vi "example.vi"() -> ()   [LabVIEW 2016]
panel:
  in  "Stream Write":i32
  out "Stream Writer Loop readback":i32
  out "Stream Reader":i32
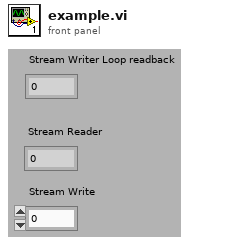
[diagram p1: front panel]
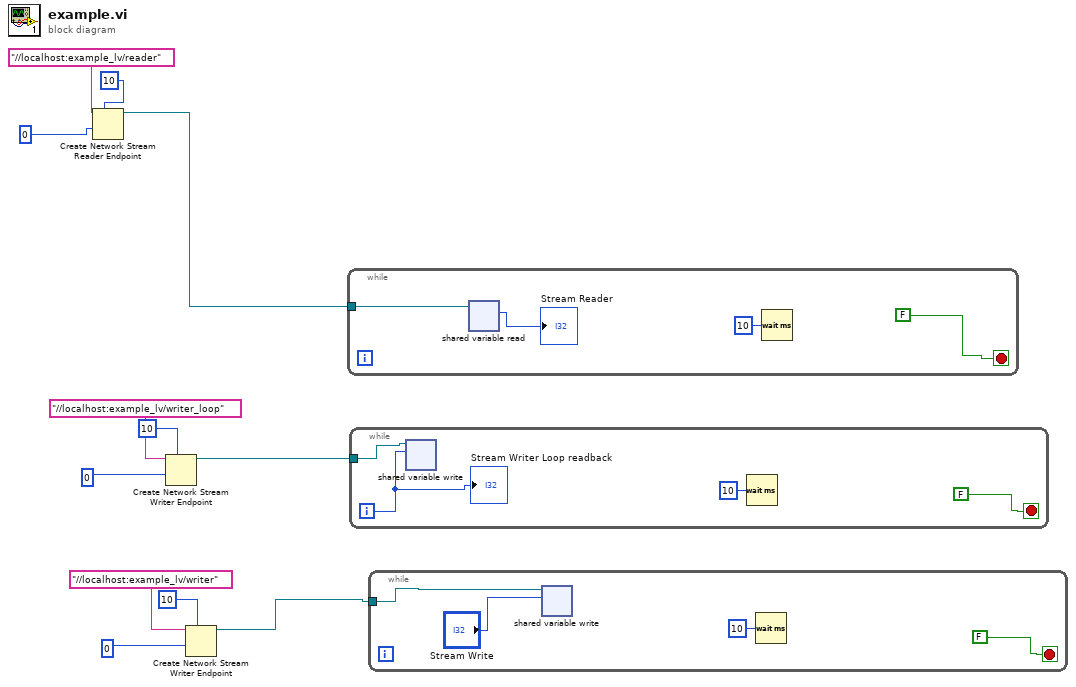
[diagram p0: block diagram]
diagram:
  n1 = Create Network Stream Reader Endpoint(7:10 ("writer buffer size"), 9:0, 11:"//localhost:example_lv/reader") -> (3:w6:refnum<k21>)  [unwired: 4 in, 1 out]
  n2 = Create Network Stream Writer Endpoint(7:10 ("writer buffer size"), 9:0, 11:"//localhost:example_lv/writer_loop") -> (3:w5:refnum<k21>)  [unwired: 4 in, 1 out]
  n3 = Create Network Stream Writer Endpoint(7:10 ("writer buffer size"), 9:0, 11:"//localhost:example_lv/writer") -> (3:w1:refnum<k21>)  [unwired: 4 in, 1 out]
  n4 = while {
    tunnel: w6 -> [w16]
    stop <- FALSE ("Some Button") stop-if-true
    n5 = shared-variable-read(w16) -> (→"Stream Reader":i32)  [unwired: 2 in, 3 out]
    n6 = Wait (ms)(milliseconds to wait=u32 10) -> ()  [unwired: 1 out]
  }
  n7 = while {
    tunnel: w5 -> [w18]
    i -> [w19]
    stop <- FALSE ("Some Button") stop-if-true
    n8 = shared-variable-write(w18, w19) -> ()  [unwired: 2 in, 3 out]
    n9 = Wait (ms)(milliseconds to wait=u32 10) -> ()  [unwired: 1 out]
    "Stream Writer Loop readback" <- w19
  }
  n10 = while {
    tunnel: w1 -> [w23]
    stop <- FALSE ("Some Button") stop-if-true
    n11 = shared-variable-write(w23, "Stream Write") -> ()  [unwired: 2 in, 3 out]
    n12 = Wait (ms)(milliseconds to wait=u32 10) -> ()  [unwired: 1 out]
  }
